vi "post_dust_event_small.vi"(8 "error in (no error)":errorcluster, 10 "Signal Array":T1[](array[typedef]), 11 "Cluster":T4 {"File Location" items=["Unknown"=-1, "Processing"=0, "Storage"=1]}) -> (0 "error out":errorcluster, 1 "Experiment Settings":i32, 2 "Dust Event ID":i32, 3 "Test Server":bool)   [LabVIEW 2013]
uses:
  Small Accelerator/Post_Dust_Event_small.ctl
  Controls/File_location.ctl
  Public API/Signal.ctl
  Controls/Role ID.ctl
  Controls/Hardware ID.ctl
  <vilib>/addons/database/Auxilliary.llb/DB Tools Cursor Type.ctl
  NaN_screening_small.vi
  <vilib>/addons/database/Connection.llb/Conn Execute.vi
  <vilib>/addons/database/Recordset.llb/Rec Fetch Recordset Data (R).vi
  <vilib>/addons/database/Recordset.llb/Rec Destroy - Connection.vi
  <vilib>/addons/database/_DB Variant To Data/Database Variant To Data.xnode
  <vilib>/addons/database/NI_Database_API.lvlib
panel:
  # "Signal"
  # "Dust Event Small"
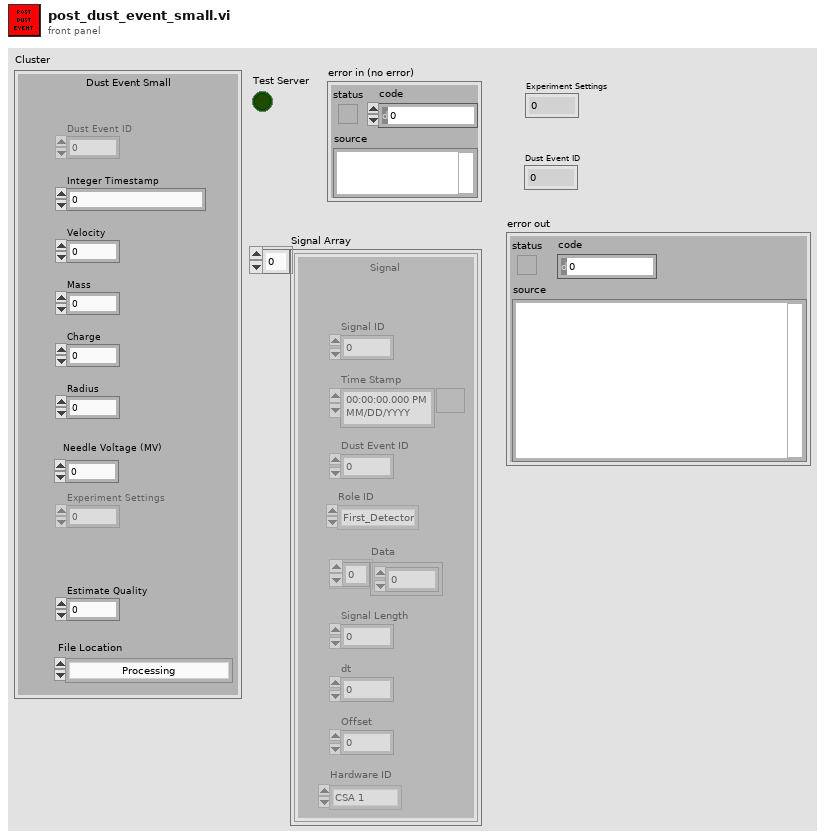
[diagram p1: front panel]
types:
  T1 = typedef "Signal.ctl" = cluster{"Signal ID":i64, "Time Stamp":timestamp, "Dust Event ID":i64, "Role ID":T2, "Data":sgl[], "Signal Length":i32, "dt":sgl, "Offset":dbl, "Hardware ID":T3}
  T2 = typedef "Role ID.ctl" = enum16{"First_Detector", "Second_Detector", "Third_Detector", "LeCroy_CH1", "LeCroy_CH2", "LeCroy_CH3", "LeCroy_CH4", "PSU"}
  T3 = typedef "Hardware ID.ctl" = enum16{"Unknown", "CSA 1", "CSA 2", "CSA 3", "CSA 4", "CSA 5", "CSA 6"}
  T4 = typedef "Post_Dust_Event_small.ctl" = cluster{"Dust Event ID":i64, "Integer Timestamp":i64, "Velocity":sgl, "Mass":sgl, "Charge":sgl, "Radius":sgl, "Needle Voltage (MV)":dbl, "Experiment Settings":dbl, "Estimate Quality":sgl, "File Location":T5, "id_dust_info":dbl}
  T5 = typedef "File_location.ctl" = i8
  T6 = typedef "NI_Database_API.lvlib/DB Tools Cursor Type.ctl" = enum16{"forward-only", "keyset", "dynamic", "static"}
  T7 = typedef "NI_Database_API.lvlib/Conn ObjectReference.ctl" = refnum<k1>
  T8 = typedef "NI_Database_API.lvlib/Rec ObjectReference.ctl" = refnum<k1>
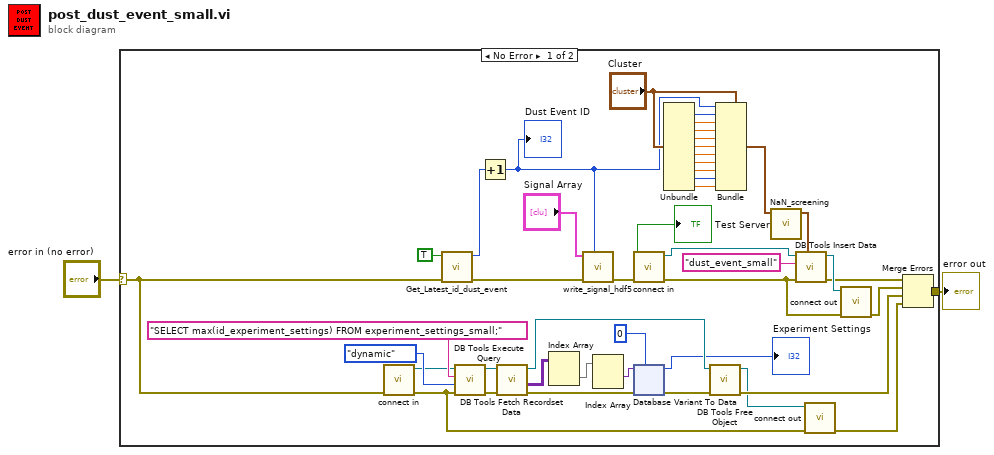
[diagram p0: block diagram]
diagram:
  n1 = case shown="No Error" "error in (no error)" {
    selector: "error in (no error)" -> [w4 w80]
    tunnel: [w46 w80] -> w1
    frame No Error {
      n2 = call "connect in.vi"("error in (no error)"=w4) -> ("error out"=w11:errorcluster, "Database Connection"=w13:T7)  [unwired: 6 in, 1 out]
      n3 = call "Get_Latest_id_dust_event.vi"("error in (no error)"=w4, "Small?"=TRUE) -> ("error out"=w6:errorcluster, "id_dust_event"=w3:i64)  [unwired: 8 in]
      n4 = call-poly <vilib>:"DB Tools Execute Query.vi"("error in (no error)"=w11, "cursor type"=DB_Tools_Cursor_Type."dynamic", "SQL query"="SELECT max(id_experiment_settings) FROM experiment_settings_small;", "connection reference"=w13) -> ("error out"=w20:errorcluster, "recordset reference"=w19:T8)  [unwired: 4 in]
      n5 = Increment(x=w3) -> (x+1=w29:i64)
      "Dust Event ID" <- w29
      n6 = call-poly <vilib>:"DB Tools Fetch Recordset Data.vi"("error in (no error)"=w20, "recordset reference"=w19) -> ("error out"=w24:errorcluster, "recordset data"=w22:variant[][], "recordset reference out"=w21:T8)  [unwired: 3 in]
      n7 = Index Array(array=w22) -> (element=w26:variant[])  [unwired: 2 in]
      n8 = call "write_signal_hdf5.vi"("Index"=w29, "error in"=w6, "Signal array"="Signal Array") -> ("error out"=w9:errorcluster)  [unwired: 7 in, 1 out]
      n9 = Index Array(array=w26) -> (element #1=w25:variant)  [unwired: 2 in, 1 out]
      n10 = call "connect in.vi"("error in (no error)"=w9) -> ("error out"=w8:errorcluster, "Database Connection"=w7:T7, "Test Server"=→"Test Server":bool)  [unwired: 6 in]
      n11 = xnode "Database Variant To Data"("database variant"=w25, "error in (no error)"=w24, "type"=0) -> ("data"=→"Experiment Settings":i32, "error out"=w27:errorcluster)
      n12 = Unbundle("Cluster") -> ("Integer Timestamp"=w30:i64, "Velocity"=w31:sgl, "Mass"=w32:sgl, "Charge"=w33:sgl, "Radius"=w34:sgl, "Needle Voltage (MV)"=w35:dbl, "Experiment Settings"=w36:dbl, "Estimate Quality"=w37:sgl, "File Location"=w28:T5, "id_dust_info"=w38:dbl)  [unwired: 1 out]
      n13 = call-poly <vilib>:"DB Tools Free Object.vi"("error in (no error)"=w27, "recordset reference"=w21) -> ("error out"=w14:errorcluster, "connection reference"=w12:T7)  [unwired: 8 in]
      n14 = Bundle(cluster="Cluster", "Dust Event ID"=w29, "Integer Timestamp"=w30, "Velocity"=w31, "Mass"=w32, "Charge"=w33, "Radius"=w34, "Needle Voltage (MV)"=w35, "Experiment Settings"=w36, "Estimate Quality"=w37, "File Location"=w28, "id_dust_info"=w38) -> (w39:T4)
      n15 = call-poly "NaN_screening.vi"("Input"=w39) -> ("Output"=w45:T4)  [unwired: 10 in]
      n16 = call <vilib>:"DB Tools Insert Data.vi"("data"=w45, "error in (no error)"=w8, "table"="dust_event_small", "connection reference"=w7) -> ("error out"=w41:errorcluster, "connection reference out"=w42:T7)  [unwired: 6 in]
      n17 = call "connect out.vi"("error in (no error)"=w11, "connection reference"=w12) -> ("error out"=w10:errorcluster)  [unwired: 9 in]
      n18 = call "connect out.vi"("error in (no error)"=w8, "connection reference"=w42) -> ("error out"=w15:errorcluster)  [unwired: 9 in]
      n19 = Merge Errors(w41, w15, w14, w10) -> (w46:errorcluster)
    }
    frame Error {
    }
  }
  "error out" <- w1
